vi "AlliGator Save ROI v3.vi"(7 "Image Label":string, 8 "Error In":errorcluster, 11 "ROI Description":T1 {"ROI Descriptor"."Contours"."Type" items=["No Selection", "Point", "Line", "Rectangle", "Oval", "Polygon", "Freehand Region", "Annulus", "Unused2", "Unused3", "Broken Line", "Freehand Line", "Rotated Rectangle"]}) -> (0 "Error Out":errorcluster, 3 "Notebook Message":string)   [LabVIEW 2021, in "AlliGator ROIs.lvlib"]
doc: "Saves single ROI."
uses:
  AlliGator ROIs.lvlib
  Image/Named ROI Description.ctl
  Image/Image Control ROI Description v2.ctl
  89dc576b-80b0-491c-980e-ed8170e4db80.vi
  <vilib>/JDP Science/JSONtext/Variant to JSON Text.vi
  <vilib>/JDP Science/JSONtext/LVClass Serializer/JSONtext LVClass Serializer.lvclass
  Image/Image.lvlib
panel:
  # "see the AlliGator License on the block diagram (Ctrl+E or Window:Show Block Diagram)"
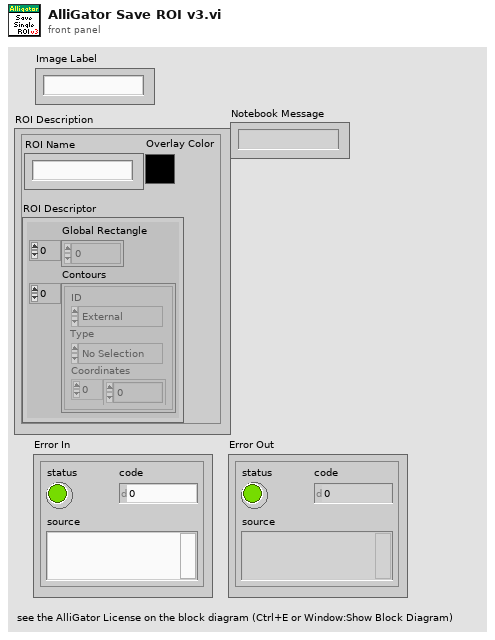
[diagram p1: front panel]
types:
  T1 = typedef "Image.lvlib/Named ROI Description.ctl" = cluster{"ROI Descriptor":T2, "ROI Name":string, "Overlay Color":u32}
  T2 = typedef "ROI Descriptor" = cluster{"Global Rectangle":i32[], "Contours":cluster{"ID":enum32{"External", "Internal"}, "Type":u32, "Coordinates":i32[]}[]}
  T3 = typedef "Image.lvlib/Image Control ROI Description v2.ctl" = cluster{"Image Control Label":string, "Named ROI Description":T1}
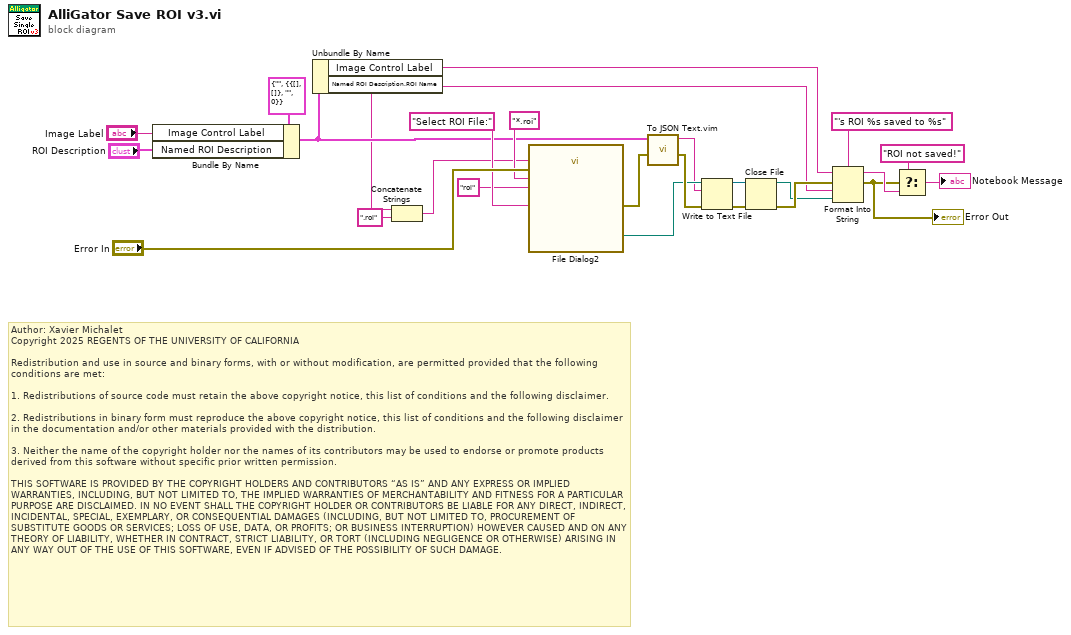
[diagram p0: block diagram]
diagram:
  # "Author: Xavier Michalet\nCopyright 2025 REGENTS OF THE UNIVERSITY OF CALIFORNIA\n\nRedistribution and use in source and binary forms, with or without modification, are permitted provided that the following conditions are met:\n\n1. Redistributions of source code must retain the above copyright notice, this list of conditions and the following disclaimer.\n\n2. Redistributions in binary form must reproduce the above copyright notice, this list of conditions and the following disclaimer in the documentation and/or other materials provided with the distribution.\n\n3. Neither the name of the copyright holder nor the names of its contributors may be used to endorse or promote products derived from this software without specific prior written permission.\n\nTHIS SOFTWARE IS PROVIDED BY THE COPYRIGHT HOLDERS AND CONTRIBUTORS “AS IS” AND ANY EXPRESS OR IMPLIED WARRANTIES, INCLUDING, BUT NOT LIMITED TO, THE IMPLIED WARRANTIES OF MERCHANTABILITY AND FITNESS FOR A PARTICULAR PURPOSE ARE DISCLAIMED. IN NO EVENT SHALL THE COPYRIGHT HOLDER OR CONTRIBUTORS BE LIABLE FOR ANY DIRECT, INDIRECT, INCIDENTAL, SPECIAL, EXEMPLARY, OR CONSEQUENTIAL DAMAGES (INCLUDING, BUT NOT LIMITED TO, PROCUREMENT OF SUBSTITUTE GOODS OR SERVICES; LOSS OF USE, DATA, OR PROFITS; OR BUSINESS INTERRUPTION) HOWEVER CAUSED AND ON ANY THEORY OF LIABILITY, WHETHER IN CONTRACT, STRICT LIABILITY, OR TORT (INCLUDING NEGLIGENCE OR OTHERWISE) ARISING IN ANY WAY OUT OF THE USE OF THIS SOFTWARE, EVEN IF ADVISED OF THE POSSIBILITY OF SUCH DAMAGE."
  n1 = Bundle By Name(cluster=T3 {"Image Control Label"="", "Named ROI Description"={"ROI Descriptor"={"Global Rectangle"=[], "Contours"=[]}, "ROI Name"="", "Overlay Color"=0}} ("Image Control ROI Description"), "Image Control Label"="Image Label", "Named ROI Description"="ROI Description") -> (w10:T3)
  n2 = Unbundle By Name(w10) -> ("Image Control Label"=w20:string, "Named ROI Description.ROI Name"=w9:string)
  n3 = Concatenate Strings(w9, ".roi" ("string")) -> (w7:string)
  n4 = call "File Dialog2"("prompt"="Select ROI File:" ("Prompt"), "default name"=w7, "error in"="Error In", "pattern (all files)"="*.roi" ("Pattern (*.xml;*.XML)"), "pattern label"="roi" ("File Extension (xml)")) -> ("selected path"=w4:path, "error out"=w6:errorcluster)  [unwired: 7 in, 2 out]
  n5 = call "To JSON Text.vim"("error in (no error)"=w6, "Anything"=w10) -> ("error out"=w5:errorcluster, "<JSON>"=w1:string)  [unwired: 8 in]
  n6 = Write to Text File(file (use dialog)=w4, text=w1, error in=w5) -> (refnum out=w3:refnum<file>, error out=w2:errorcluster)  [unwired: 1 in, 1 out]
  n7 = Close File(refnum=w3, error in=w2) -> (path=w14:path, error out=w22:errorcluster)
  n8 = Format Into String(format string="'s ROI %s saved to %s", initial string=w20, error in=w22, w9, w14) -> (resulting string=w23:string, error out=w18:errorcluster)
  "Error Out" <- w18
  n9 = Select(t="ROI not saved!", s=w18, f=w23) -> (s? t:f=→"Notebook Message":string)
